vi "2_to_2-10.vi"(1 "input":T2) -> (0 "output":T1)   [LabVIEW 2013]
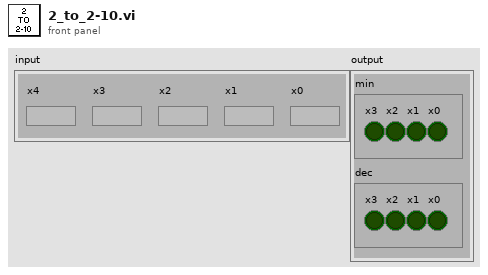
[diagram p1: front panel]
types:
  T1 = cluster{"min":cluster{"x3":bool, "x2":bool, "x1":bool, "x0":bool}, "dec":cluster{"x3":bool, "x2":bool, "x1":bool, "x0":bool}}
  T2 = cluster{"x4":bool, "x3":bool, "x2":bool, "x1":bool, "x0":bool}
  T3 = cluster{cluster{"S":bool, "S":bool, "S":bool, "S":bool}, cluster{"C":bool, "S":bool, "S":bool, "S":bool}}
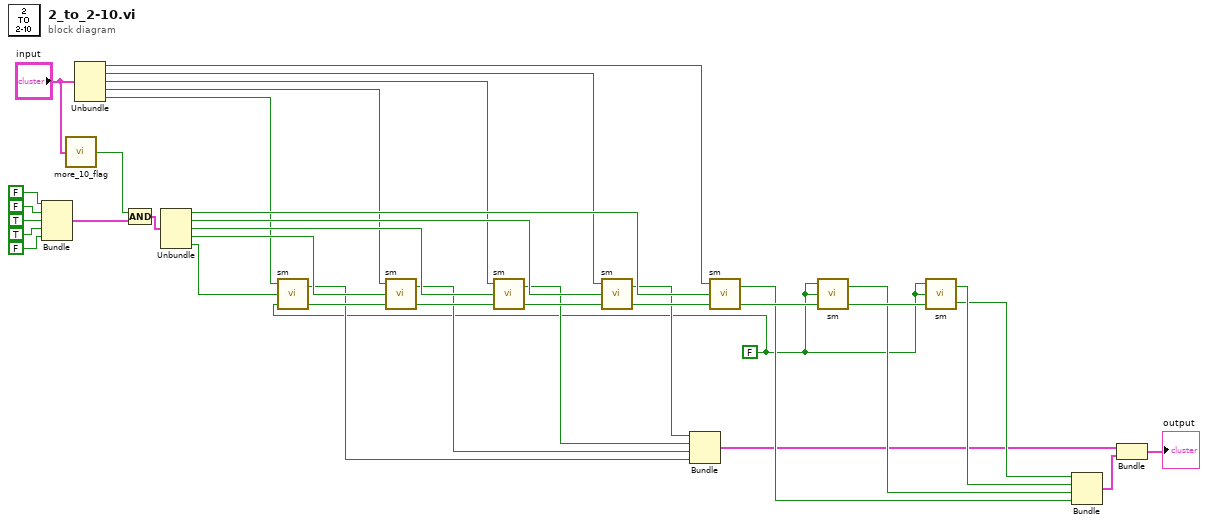
[diagram p0: block diagram]
diagram:
  w1 = FALSE
  n1 = Bundle(FALSE, FALSE, TRUE, TRUE, FALSE) -> (w32:cluster{bool, bool, bool, bool, bool})  [unwired: 1 in]
  n2 = call "more_10_flag.vi"("input"="input") -> ("flag"=w31:bool)
  n3 = Unbundle("input") -> ("x4"=w20:bool, "x3"=w21:bool, "x2"=w22:bool, "x1"=w24:bool, "x0"=w23:bool)
  n4 = Compound Arithmetic op=AND(w31, w32) -> (w30:cluster{bool, bool, bool, bool, bool})
  n5 = Unbundle(w30) -> (w25:bool, w26:bool, w27:bool, w28:bool, w29:bool)
  n6 = call "sm.vi"("c"=w1, "b"=w29, "a"=w23) -> ("C"=w19:bool, "S"=w12:bool)
  n7 = call "sm.vi"("c"=w19, "b"=w28, "a"=w24) -> ("C"=w18:bool, "S"=w11:bool)
  n8 = call "sm.vi"("c"=w18, "b"=w27, "a"=w22) -> ("C"=w17:bool, "S"=w10:bool)
  n9 = call "sm.vi"("c"=w17, "b"=w26, "a"=w21) -> ("C"=w16:bool, "S"=w9:bool)
  n10 = Bundle("S"=w9, "S"=w10, "S"=w11, "S"=w12) -> (w3:cluster{"S":bool, "S":bool, "S":bool, "S":bool})  [unwired: 1 in]
  n11 = call "sm.vi"("c"=w16, "b"=w25, "a"=w20) -> ("C"=w15:bool, "S"=w8:bool)
  n12 = call "sm.vi"("c"=w15, "b"=w1, "a"=w1) -> ("C"=w14:bool, "S"=w7:bool)
  n13 = call "sm.vi"("c"=w14, "b"=w1, "a"=w1) -> ("C"=w5:bool, "S"=w6:bool)
  n14 = Bundle("C"=w5, "S"=w6, "S"=w7, "S"=w8) -> (w4:cluster{"C":bool, "S":bool, "S":bool, "S":bool})  [unwired: 1 in]
  n15 = Bundle(w3, w4) -> (→"output":T3)  [unwired: 1 in]
